vi "报警值接收解析.vi"(11 "完整输入":string="\u0001\u0003\u0004\u0014\u0000\u0000\u0000ÿÃ") -> (1 "有效数据？":bool, 3 "限值":dbl)   [LabVIEW 2017]
panel:
  out "探头号":u16
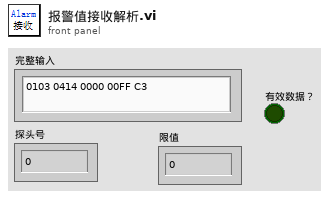
[diagram p1: front panel]
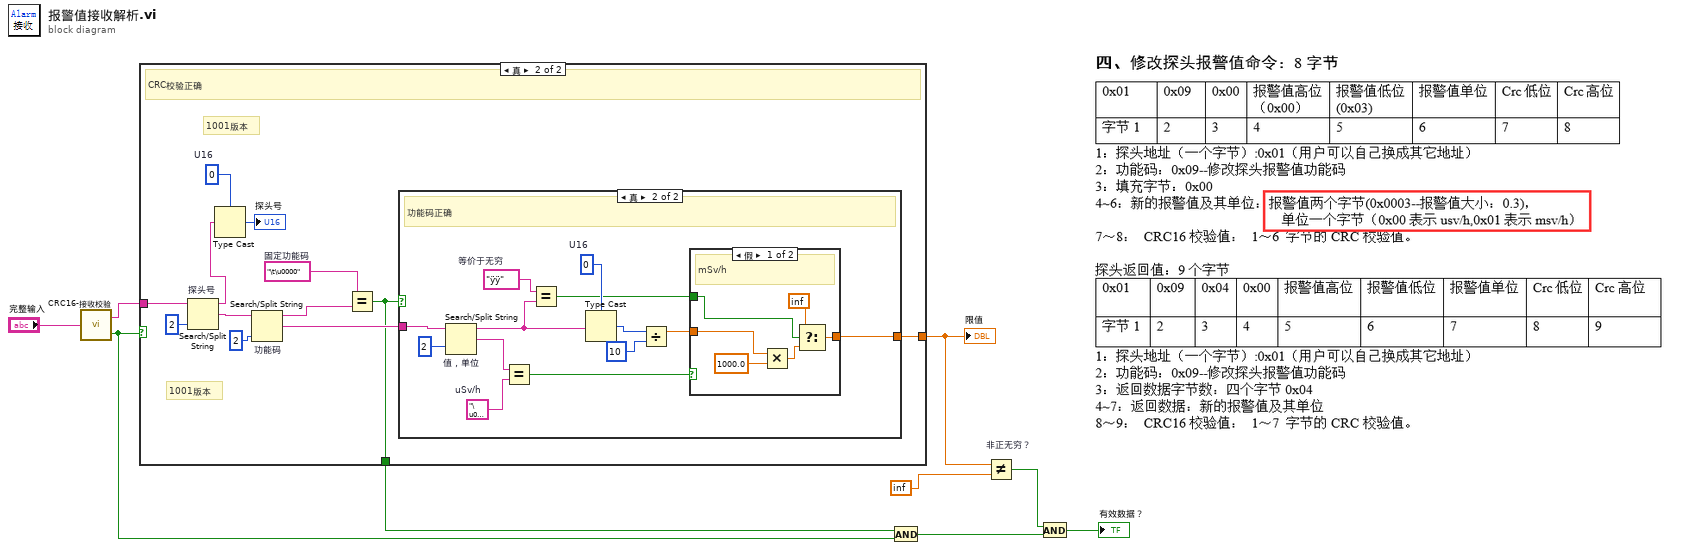
[diagram p0: block diagram]
diagram:
  n1 = call "CRC16-接收校验.vi"("读取缓冲区"="完整输入") -> ("净数据"=w8:string, "CRC？"=w7:bool)
  n2 = case shown="真" w7 {
    tunnel: w8 -> [_ w15]
    tunnel: [_ w19] -> w3
    tunnel: [_ w10] -> w6
    frame False {
    }
    frame True {
      w13 = u16 0  # U16
      w17 = "\t\u0000"  # 固定功能码
      # "1001版本"
      # "1001版本"
      # "CRC校验正确"
      n3 = Search/Split String "探头号"(string=w15, offset (0)=2 ("偏移量(0)")) -> (substring before match=w12:string, match + rest of string=w14:string)  [unwired: 1 in, 1 out]
      n4 = Type Cast(type=w13, x=w12) -> (*(type *) &x=→"探头号":u16)
      n5 = Search/Split String "功能码"(string=w14, offset (0)=2 ("偏移量(0)")) -> (substring before match=w18:string, match + rest of string=w20:string)  [unwired: 1 in, 1 out]
      n6 = Equal?(x=w17, y=w18) -> (x = y?=w10:bool)
      n7 = case shown="真" w10 {
        tunnel: w20 -> [_ w34]
        tunnel: [_ w28] -> w19
        frame False {
          # "功能码错误"
        }
        frame True {
          w23 = "ÿÿ"  # 等价于无穷
          w30 = "\u0000"  # uSv/h
          w32 = u16 0  # U16
          # "功能码正确"
          n8 = Search/Split String "值，单位"(string=w34, offset (0)=2 ("偏移量(0)")) -> (substring before match=w24:string, match + rest of string=w31:string)  [unwired: 1 in, 1 out]
          n9 = Equal?(x=w31, y=w30) -> (x = y?=w29:bool)
          n10 = Equal?(x=w23, y=w24) -> (x = y?=w22:bool)
          n11 = Type Cast(type=w32, x=w24) -> (*(type *) &x=w27:u16)
          n12 = Divide(x=w27, y=u16 10) -> (x/y=w26:dbl)
          n13 = case shown="假" w29 {
            tunnel: w26 -> [w40 w41]
            tunnel: [w35 w41] -> w28
            tunnel: w22 -> [w38 _]
            frame False {
              # "mSv/h"
              n14 = Multiply(x=w40, y=1000.0) -> (x*y=w36:dbl)
              n15 = Select(t=inf, s=w38, f=w36) -> (s? t:f=w35:dbl)
            }
            frame True {
              # "uSv/h"
            }
          }
        }
      }
    }
  }
  "限值" <- w3
  n16 = And(x=w6, y=w7) -> (x .and. y?=w5:bool)
  n17 = Not Equal? "非正无穷？"(x=w3, y=inf) -> (x != y?=w1:bool)
  n18 = And(x=w1, y=w5) -> (x .and. y?=→"有效数据？":bool)
